vi "NR Fetch CHP.vi"(0 "RFmx Handle In":refnum<k21>, 1 "Selector String":string, 11 "error in (no error)":errorcluster) -> (4 "RFmx Handle Out":refnum<k21>, 6 "CHP Results":T1, 15 "error out":errorcluster)   [LabVIEW 2016, in "RFmxNR.lvlib"]
doc: "Fetches common results from the CHP measurement."
uses:
  RFmxNR.lvlib
  Typedefs/NR CHP Results.ctl
  Typedefs/NR CHP Component Carrier Results.ctl
  <vilib>/RFmx/NR/mx/RFmxNR.llb/RFmxNR CHP Fetch Total Aggregated Power.vi
  <vilib>/RFmx/NR/mx/RFmxNR.llb/RFmxNR CHP Fetch Component Carrier Measurement (Array).vi
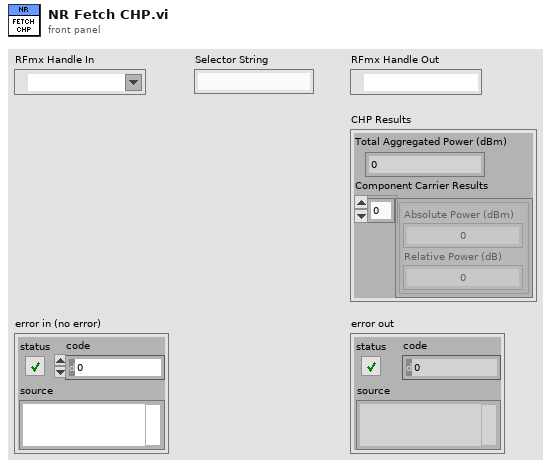
[diagram p1: front panel]
types:
  T1 = typedef "RFmxNR.lvlib/NR CHP Results.ctl" = cluster{"Total Aggregated Power (dBm)":dbl, "Component Carrier Results":T2[]}
  T2 = typedef "RFmxNR.lvlib/NR CHP Component Carrier Results.ctl" = cluster{"Absolute Power (dBm)":dbl, "Relative Power (dB)":dbl}
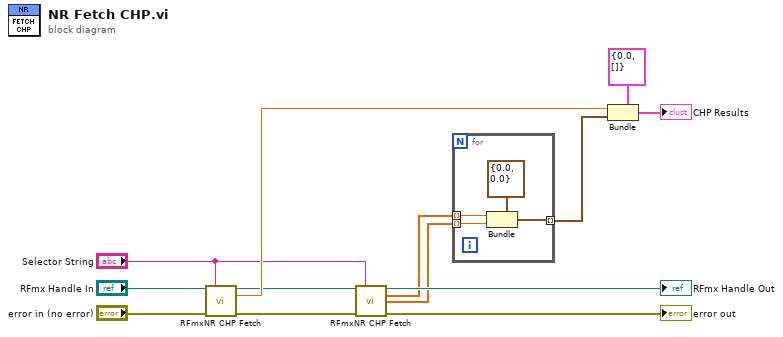
[diagram p0: block diagram]
diagram:
  n1 = call-poly <vilib>:"RFmxNR CHP Fetch.vi"("Instrument Handle In"="RFmx Handle In", "Selector String"="Selector String", "error in (no error)"="error in (no error)") -> ("Instrument Handle Out"=w9:refnum<k21>, "Total Aggregated Power (dBm)"=w10:dbl, "error out"=w8:errorcluster)  [unwired: 10 in]
  n2 = call-poly <vilib>:"RFmxNR CHP Fetch.vi"("Instrument Handle In"=w9, "Selector String"="Selector String", "error in (no error)"=w8) -> ("Instrument Handle Out"=→"RFmx Handle Out":refnum<k21>, "Absolute Power (dBm)"=w4:dbl[], "Relative Power (dB)"=w3:dbl[], "error out"=→"error out":errorcluster)  [unwired: 9 in]
  n3 = for {
    tunnel: w4 -> [w16] mode=indexing
    tunnel: w3 -> [w15] mode=indexing
    tunnel: [w14] -> w2 mode=indexing
    n4 = Bundle(cluster=T2 {"Absolute Power (dBm)"=0.0, "Relative Power (dB)"=0.0} ("NR CHP Component Carrier Results"), "Absolute Power (dBm)"=w16, "Relative Power (dB)"=w15) -> (w14:T2)
  }
  n5 = Bundle(cluster=T1 {"Total Aggregated Power (dBm)"=0.0, "Component Carrier Results"=[]} ("NR CHP Results"), "Total Aggregated Power (dBm)"=w10, "Component Carrier Results"=w2) -> (→"CHP Results":T1)
